vi "TWM Get Session Parameters.vi"(8 "error in":errorcluster, 11 "meas root":path) -> (0 "error out":errorcluster, 2 "TWM session data":string, 3 "TWM session items":T1)   [LabVIEW 2013]
doc: "Retrieves TWM measurement session file and parses some of the parameters."
uses:
  TWM Session Data.ctl
  <vilib>/Analysis/baseanly.llb/Mean (DBL).vi
  infolib.lvlibp/Private/Get matrix polymorph parts/Get 1D String.vi
  infolib.lvlibp/Private/Get matrix polymorph parts/Get 1D EXT.vi
  infolib.lvlibp/Private/Get matrix polymorph parts/Get 1D I64.vi
  infolib.lvlibp/Private/Get matrix polymorph parts/Get 2D I64.vi
  infolib.lvlibp/Private/Get key polymorph parts/GetString.vi
  infolib.lvlibp
  <vilib>/Analysis/NI_AALBase.lvlib
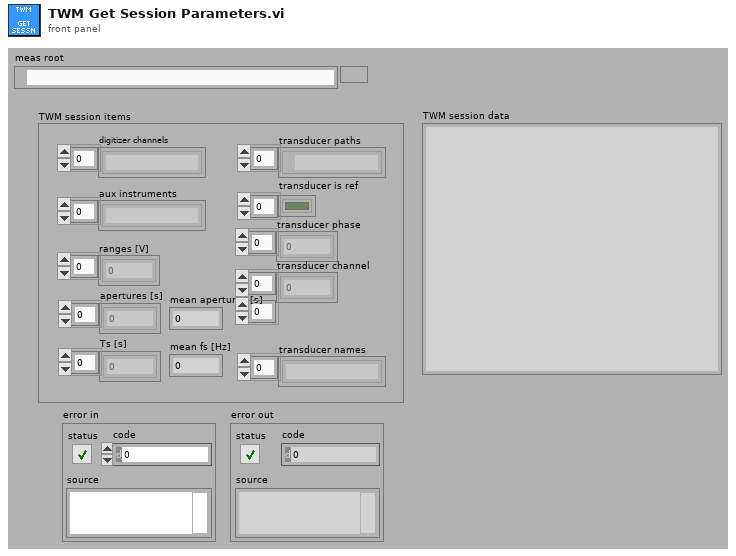
[diagram p1: front panel]
types:
  T1 = typedef "TWM Session Data.ctl" = cluster{"digitizer channels":string[], "aux instruments":string[], "ranges [V]":dbl[], "apertures [s]":dbl[], "Ts [s]":dbl[], "mean apertures [s]":dbl, "mean fs [Hz]":dbl, "transducer paths":path[], "transducer is ref":bool[], "transducer phase":i32[], "transducer channel":i32[][], "transducer names":string[]}
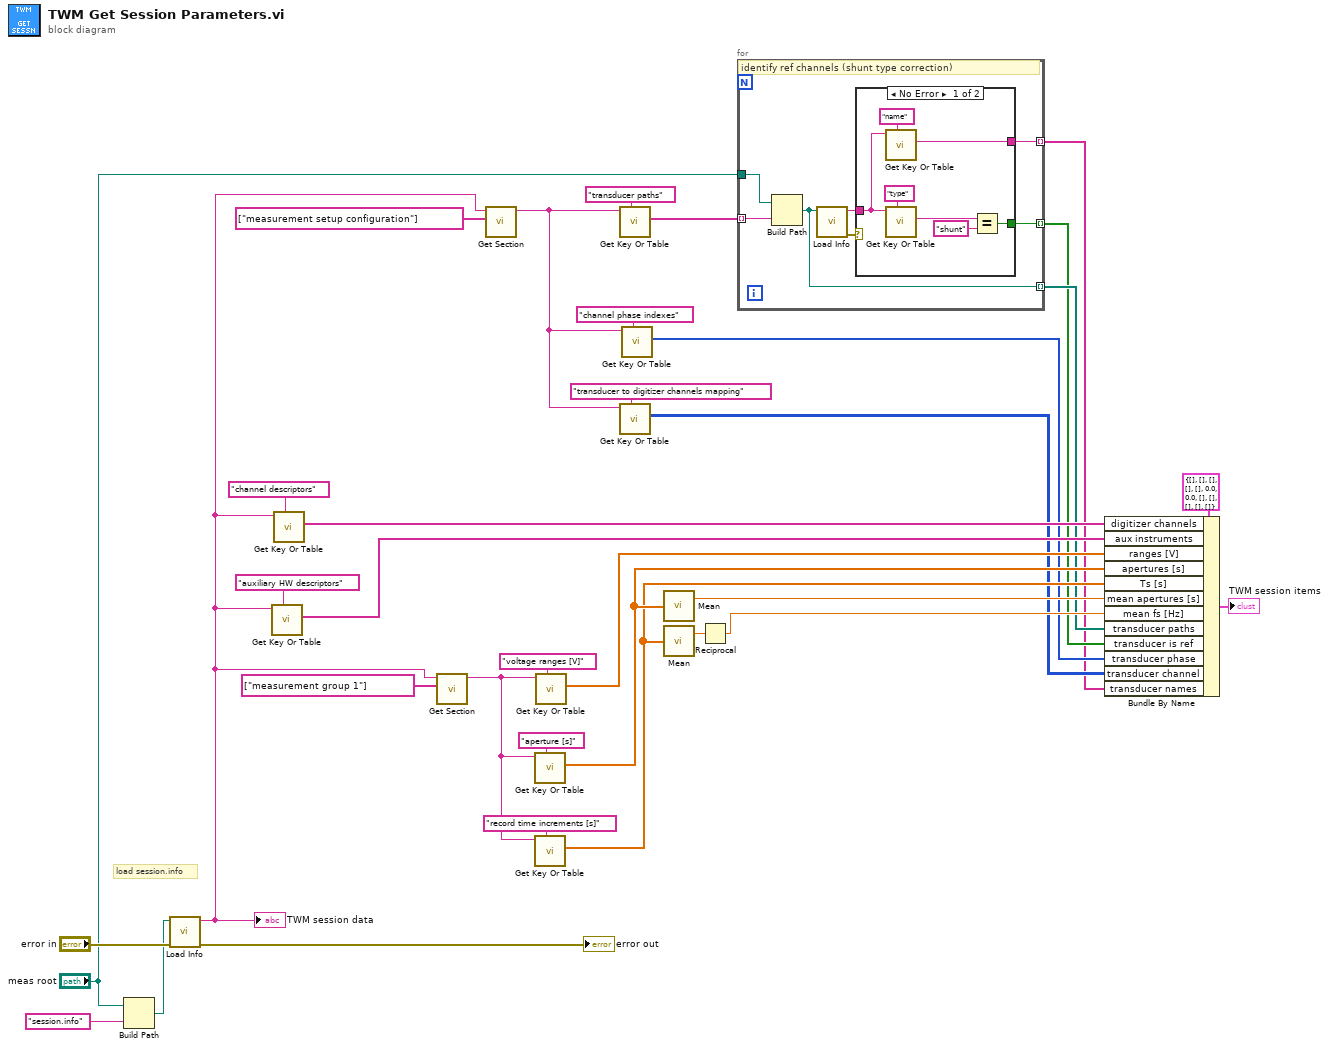
[diagram p0: block diagram]
diagram:
  # "load session.info"
  n1 = Build Path(base path="meas root", name or relative path="session.info") -> (appended path=w32:path)
  n2 = call "Load Info.vi"("error in"="error in", "filename"=w32) -> ("error out"=→"error out":errorcluster, "info data"=w13:string)  [unwired: 8 in]
  "TWM session data" <- w13
  n3 = call-poly "Get Key Or Table.vi"("key description"="auxiliary HW descriptors", "info data"=w13) -> ("value"=w22:string[])  [unwired: 6 in, 3 out]
  n4 = call-poly "Get Key Or Table.vi"("key description"="channel descriptors", "info data"=w13) -> ("value"=w23:string[])  [unwired: 6 in, 3 out]
  n5 = call "Get Section.vi"("sections"=string[] ["measurement group 1"], "info data"=w13) -> ("section part"=w25:string)  [unwired: 8 in, 1 out]
  n6 = call "Get Section.vi"("sections"=string[] ["measurement setup configuration"], "info data"=w13) -> ("section part"=w9:string)  [unwired: 8 in, 1 out]
  n7 = call-poly "Get Key Or Table.vi"("key description"="aperture [s]", "info data"=w25) -> ("value"=w20:ext[])  [unwired: 6 in, 3 out]
  n8 = call-poly "Get Key Or Table.vi"("key description"="record time increments [s]", "info data"=w25) -> ("value"=w18:ext[])  [unwired: 6 in, 3 out]
  n9 = call-poly "Get Key Or Table.vi"("key description"="voltage ranges [V]", "info data"=w25) -> ("value"=w21:ext[])  [unwired: 6 in, 3 out]
  n10 = call-poly "Get Key Or Table.vi"("key description"="transducer paths", "info data"=w9) -> ("value"=w8:string[])  [unwired: 6 in, 3 out]
  n11 = call-poly "Get Key Or Table.vi"("key description"="transducer to digitizer channels mapping", "info data"=w9) -> ("value"=w3:i64[][])  [unwired: 6 in, 3 out]
  n12 = call-poly "Get Key Or Table.vi"("key description"="channel phase indexes", "info data"=w9) -> ("value"=w4:i64[])  [unwired: 6 in, 3 out]
  n13 = call-poly <vilib>:"Mean.vi"("X"=w20) -> ("mean"=w19:dbl)  [unwired: 1 out]
  n14 = call-poly <vilib>:"Mean.vi"("X"=w18) -> ("mean"=w17:dbl)  [unwired: 1 out]
  n15 = Reciprocal(x=w17) -> (1/x=w16:dbl)
  n16 = for {
    tunnel: w8 -> [w41] mode=indexing
    tunnel: "meas root" -> [w40]
    tunnel: [w37] -> w5 mode=indexing
    tunnel: [w36] -> w6 mode=indexing
    tunnel: [w35] -> w1 mode=indexing
    # "identify ref channels (shunt type correction)"
    n17 = Build Path(base path=w40, name or relative path=w41) -> (appended path=w36:path)
    n18 = call "Load Info.vi"("filename"=w36) -> ("error out"=w38:errorcluster, "info data"=w39:string)  [unwired: 9 in]
    n19 = case shown="No Error" w38 {
      tunnel: w39 -> [w43 _]
      tunnel: [w45 _] -> w37
      tunnel: [w42 _] -> w35
      frame No Error {
        n20 = call-poly "Get Key Or Table.vi"("key description"="name", "info data"=w43) -> ("value"=w42:string)  [unwired: 6 in, 3 out]
        n21 = call-poly "Get Key Or Table.vi"("key description"="type", "info data"=w43) -> ("value"=w47:string)  [unwired: 6 in, 3 out]
        n22 = Equal?(x=w47, y="shunt") -> (x = y?=w45:bool)
      }
      frame Error {
      }
    }
  }
  n23 = Bundle By Name(cluster=T1 {"digitizer channels"=[], "aux instruments"=[], "ranges [V]"=[], "apertures [s]"=[], "Ts [s]"=[], "mean apertures [s]"=0.0, "mean fs [Hz]"=0.0, "transducer paths"=[], "transducer is ref"=[], "transducer phase"=[], "transducer channel"=[], "transducer names"=[]} ("TWM session items"), "digitizer channels"=w23, "aux instruments"=w22, "ranges [V]"=w21, "apertures [s]"=w20, "Ts [s]"=w18, "mean apertures [s]"=w19, "mean fs [Hz]"=w16, "transducer paths"=w6, "transducer is ref"=w5, "transducer phase"=w4, "transducer channel"=w3, "transducer names"=w1) -> (→"TWM session items":T1)
